vi "Aim drawings.vi"(1 "Particle Scores":T2, 2 "Processed Image":T1(plugin-control), 3 "Needed to show height":dbl, 4 "Center target position real life height":dbl, 5 "Center target position Y":dbl, 6 "Y ratio":dbl) -> (0 "Processed Image + aim markings":T1(plugin-control))   [LabVIEW 2012]
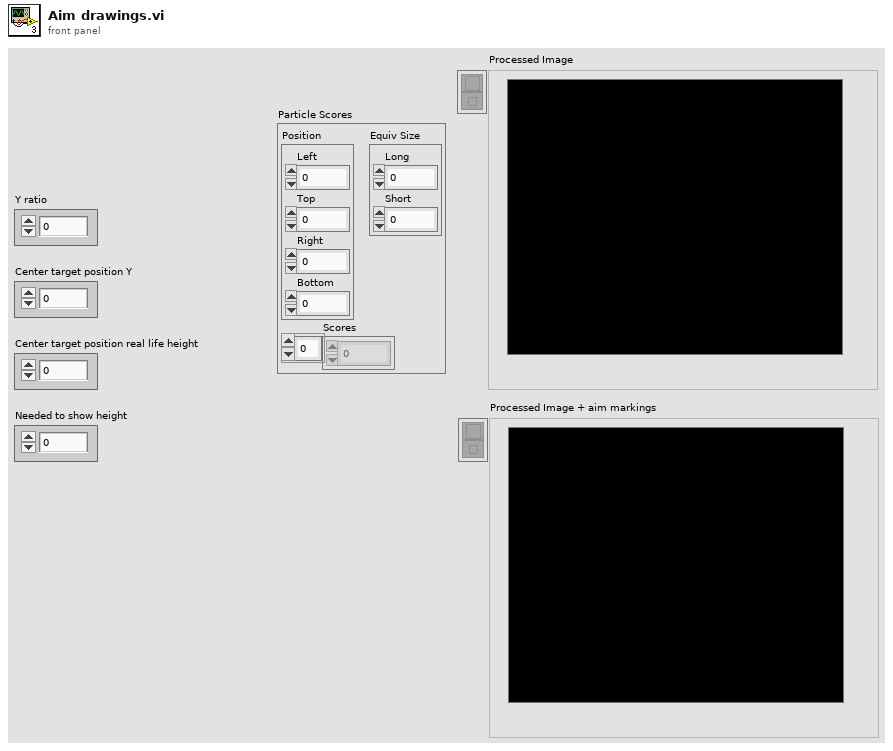
[diagram p1: front panel]
types:
  T1 = typedef "IMAQ Image.ctl" = refnum<image>
  T2 = cluster{"Position":cluster{"Left":dbl, "Top":dbl, "Right":dbl, "Bottom":dbl}, "Scores":dbl[], "Equiv Size":cluster{"Long":dbl, "Short":dbl}}
  T3 = cluster{"Left":dbl, "Top":dbl, "Right":dbl, "Bottom":dbl}
  T4 = cluster{"Left":i32, "Top":i32, "Right":i32, "Bottom":i32}
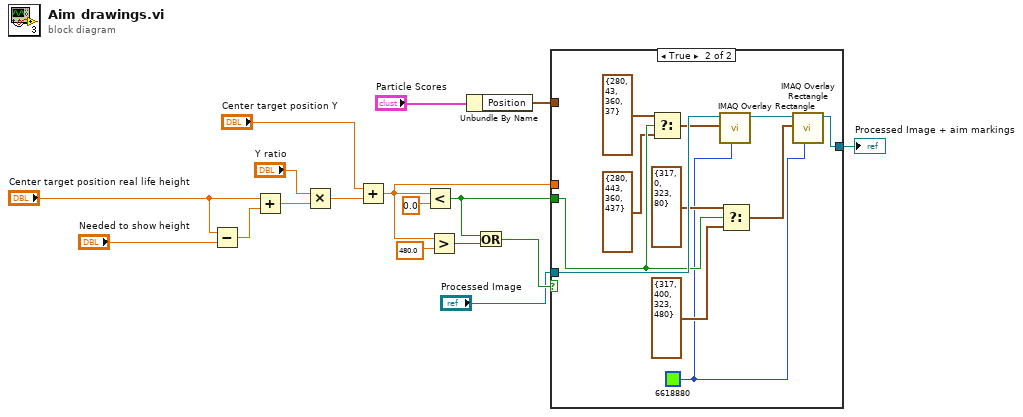
[diagram p0: block diagram]
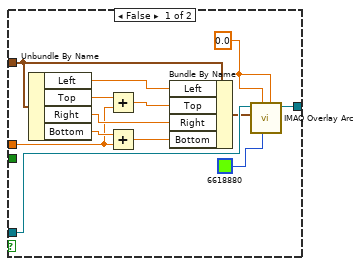
[diagram p2: hidden frame]
diagram:
  n1 = Subtract(x="Center target position real life height", y="Needed to show height") -> (x-y=w16:dbl)
  n2 = Add(x="Center target position real life height", y=w16) -> (x+y=w14:dbl)
  n3 = Multiply(x="Y ratio", y=w14) -> (x*y=w7:dbl)
  n4 = Add(x="Center target position Y", y=w7) -> (x+y=w1:dbl)
  n5 = Less?(x=w1, y=0.0) -> (x < y?=w5:bool)
  n6 = Greater?(x=w1, y=480.0) -> (0:w9:bool)
  n7 = Unbundle By Name("Particle Scores") -> ("Position"=w2:T3)
  n8 = Or(x=w5, y=w9) -> (x .or. y?=w11:bool)
  n9 = case shown="True" w11 {
    tunnel: w5 -> [_ w38]
    tunnel: [w19 w40] -> w4
    tunnel: "Processed Image" -> [w29 w39]
    tunnel: w2 -> [w26 _]
    tunnel: w1 -> [w23 _]
    frame False {
      w30 = 0.0 ("End Angle (degrees)")
      n10 = Unbundle By Name(w26) -> ("Left"=w25:dbl, "Top"=w27:dbl, "Right"=w24:dbl, "Bottom"=w28:dbl)
      n11 = Add(x=w27, y=w23) -> (x+y=w21:dbl)
      n12 = Add(x=w28, y=w23) -> (x+y=w22:dbl)
      n13 = Bundle By Name(cluster=w26, "Left"=w25, "Top"=w21, "Right"=w24, "Bottom"=w22) -> (w20:T3)
      n14 = call "IMAQ Overlay Arc"("End Angle (degrees)"=w30, "Color"=u32 6618880, "Start Angle (degrees)"=w30, "Bounding Rectangle"=w20, "Image"=w29) -> ("Image Out"=w19:T1)  [unwired: 5 in, 1 out]
    }
    frame True {
      w31 = u32 6618880 ("Color")
      n15 = Select(t=T4 {"Left"=280, "Top"=43, "Right"=360, "Bottom"=37} ("Rectangle"), s=w38, f=T4 {"Left"=280, "Top"=443, "Right"=360, "Bottom"=437} ("Rectangle")) -> (s? t:f=w33:T4)
      n16 = call "IMAQ Overlay Rectangle"("Color"=w31, "Rectangle"=w33, "Image"=w39) -> ("Image Out"=w41:T1)  [unwired: 7 in, 1 out]
      n17 = Select(t=T4 {"Left"=317, "Top"=0, "Right"=323, "Bottom"=80} ("Rectangle"), s=w38, f=T4 {"Left"=317, "Top"=400, "Right"=323, "Bottom"=480} ("Rectangle")) -> (s? t:f=w32:T4)
      n18 = call "IMAQ Overlay Rectangle"("Color"=w31, "Rectangle"=w32, "Image"=w41) -> ("Image Out"=w40:T1)  [unwired: 7 in, 1 out]
    }
  }
  "Processed Image + aim markings" <- w4
